vi "Tosca-Analog Input Thread.vi"() -> ()   [LabVIEW 2020]
uses:
  Typedefs/Tosca-AI Live Controls.ctl
  Typedefs/Tosca-AI Stream Controls.ctl
  Typedefs/Tosca-AI UI State.ctl
  Typedefs/Tosca-AI Plot Properties.ctl
  Typedefs/Tosca-AI Control Queue Data.ctl
  Typedefs/Tosca-AI.ctl
  epl-vi-lib/TCP VIs/TCP Params.ctl
  epl-vi-lib/PXI DAQ VIs/AIDI/Typedefs/AIDI-Action.ctl
  62174e53-180b-4f65-acbd-20ff4249b710.vi
  epl-vi-lib/Utility VIs/Comparison VIs/Arrays Equal (STR).vi
  Sub VIs/Tosca-Globals.vi
panel:
  out "Digital":dbl[][](graph)
  in  "More":bool=TRUE
  out "Analog":dbl[][](graph)
  in  "Trace":bool=TRUE caption="All"
  in  "Vscale":dbl=1e-09 min=1e-09 max=10.0 format="%.0pV"
  in  "Stack":bool
  in  "Vscale":bool
  out "Load":dbl(slide) caption="5 ms" scale=0.0..1.0
  in  "Status":string
  out "scale":dbl format="1div = %.0ps"
  out "recording":bool
  in  "stream":T1
  in  "Record":bool
  in  "live":T2
  in  "finished":errorcluster
  in  "History (s)":dbl=5.0
  in  "T (ms)":dbl=500.0 caption="Frame size (ms)"
  in  "Legend":i32(listbox)
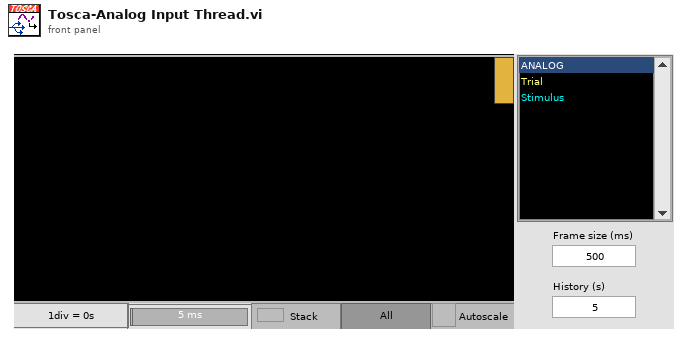
[diagram p1: front panel]
types:
  T1 = typedef "Tosca-AI Stream Controls.ctl" = cluster{"record":bool, "stem":string}
  T2 = typedef "Tosca-AI Live Controls.ctl" = cluster{"Global":cluster{"stack":bool, "auto":bool, "max":dbl}, "DI":bool[], "AI":cluster{"visible":bool, "auto":bool, "max":dbl}[], "plot AI":bool, "plot DI":bool}
  T3 = typedef "TCP Params.ctl" = cluster{"IP Address":string, "Port":i32}
  T4 = typedef "Tosca-AI.ctl" = cluster{"active":bool, "Fs":dbl, "AI":string[], "DI":string[]}
  T5 = typedef "Tosca-AI Control Queue Data.ctl" = cluster{"AI":T4, "History (s)":dbl, "T (ms)":dbl}
  T6 = typedef "Tosca-AI UI State.ctl" = cluster{"map":T7[], "running":bool, "locked":bool, "Global":cluster{"stack":bool, "auto":bool, "max":dbl}, "SelAI":i32, "first AI":i32, "plot AI":bool, "plot DI":bool, "next":string}
  T7 = typedef "Tosca-AI Plot Properties.ctl" = cluster{"graph":refnum<vi>, "plot":i32, "color":u32, "auto":bool, "visible":bool, "name":string, "digital?":bool, "max":dbl}
  T8 = cluster{"Run":refnum<user-event>, "Record":refnum<user-event>, "Stop":refnum<user-event>}
  T9 = enum8{"Enabled", "Disabled", "Disabled and Grayed Out"}
  T10 = enum16{"Sticks Top/Left", "Sticks Bottom/Right", "Proportional"}
  T11 = typedef "LVPoint32TypeDef.ctl" = cluster{"Horizontal":i32, "Vertical":i32}
  T12 = cluster{"AI":T4, "History (s)":dbl, "T (ms)":dbl}
  T13 = typedef "AIDI-Action.ctl" = enum16{"Configure", "Initialize", "Start", "Read", "Clean up", "Init & Start", "Config & Test", "Position", "Skip"}
  T14 = typedef "Tosca-AI Plot State.ctl" = cluster{"offset":i32, "nseg":i32, "nblank":i32, "npts":i32, "AI max":dbl[][], "stream":bool, "filename":string, "filenum":i32, "indicator":i32, "last ind":bool, "dig ind":bool, "nstream":i32, "istream":i32, "file":refnum<file>, "AI order":i32[], "DI order":i32[]}
  T15 = cluster{"Elapsed time (ms)":dbl, "filename":string}
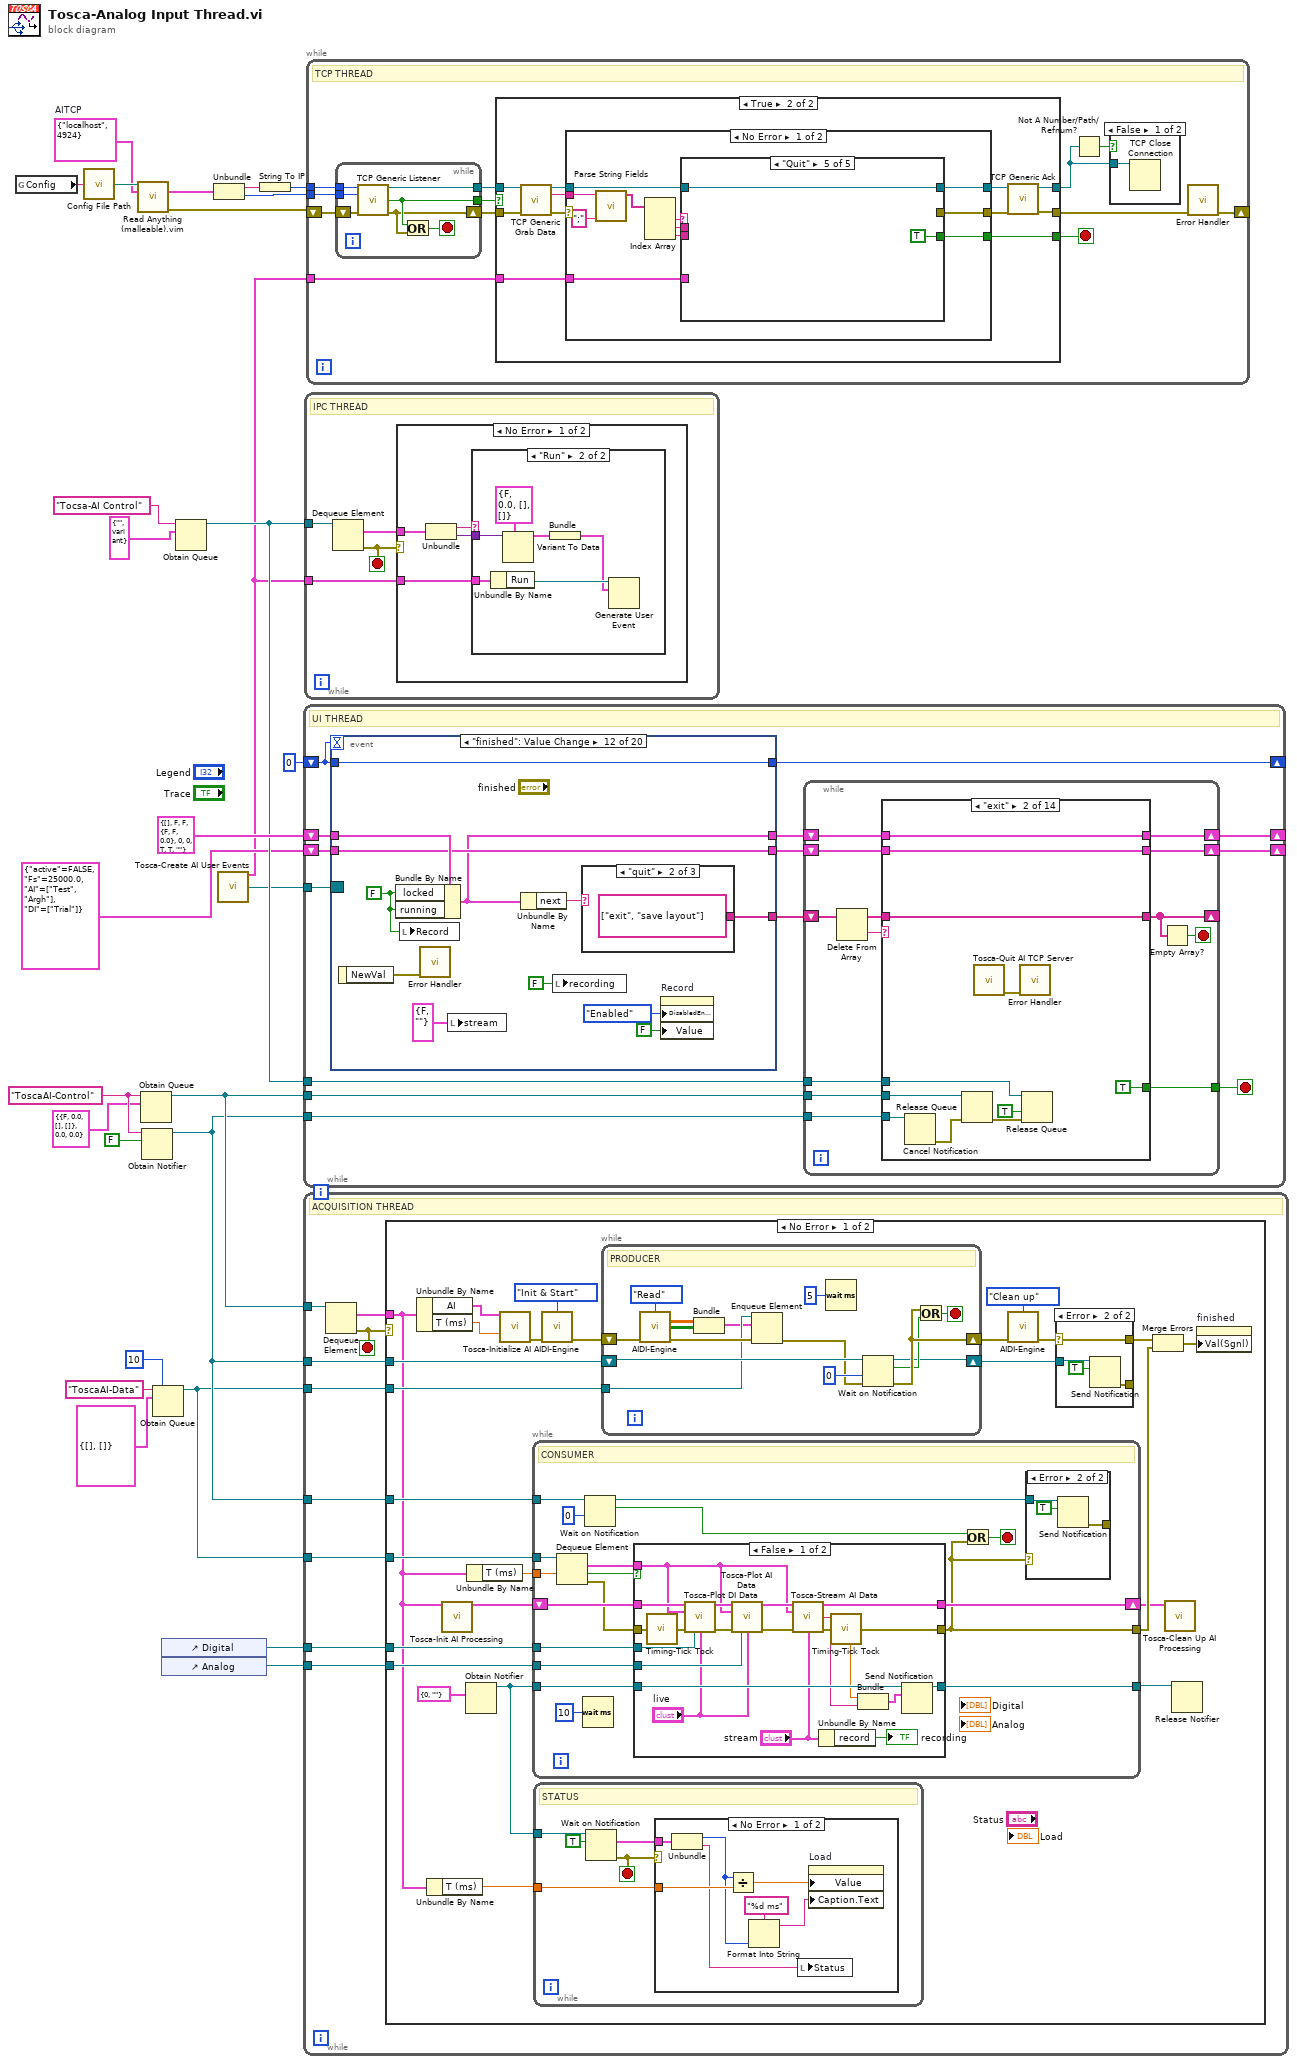
[diagram p0: block diagram]
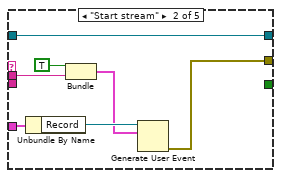
[diagram p5: hidden frame]
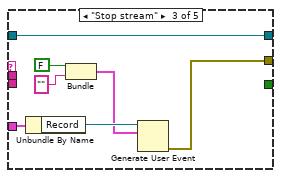
[diagram p6: hidden frame]
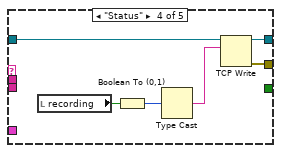
[diagram p7: hidden frame]
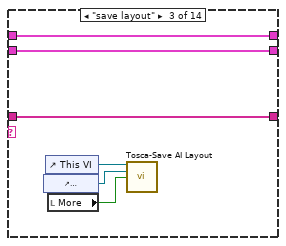
[diagram p12: hidden frame]
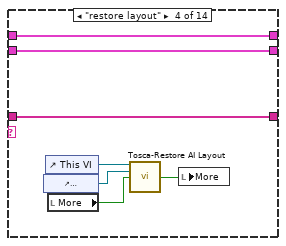
[diagram p13: hidden frame]
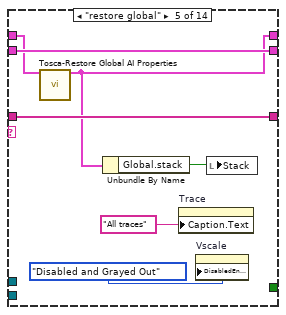
[diagram p14: hidden frame]
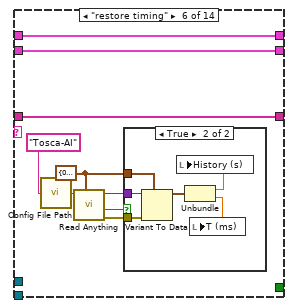
[diagram p15: hidden frame]
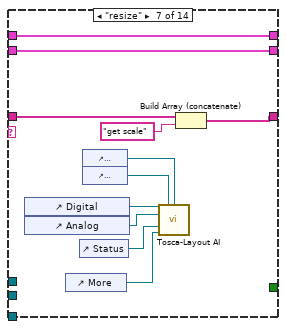
[diagram p17: hidden frame]
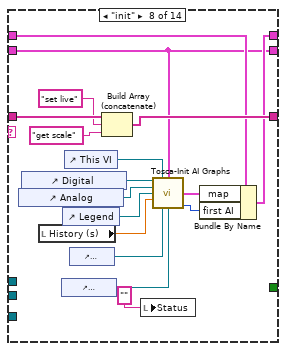
[diagram p18: hidden frame]
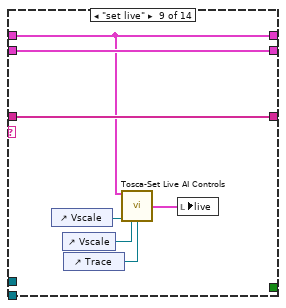
[diagram p19: hidden frame]
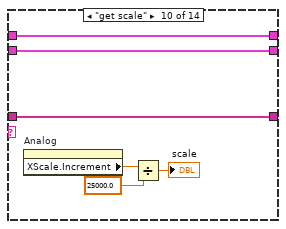
[diagram p20: hidden frame]
diagram:
  w3 = T3 {"IP Address"="localhost", "Port"=4924}  # AITCP
  w24 = "ToscaAI-Control" ("name (unnamed)")
  n1 = global read "Tosca-Globals.vi" "Config"() -> (w5:string)
  n2 = call "Config File Path.vi"("AppName"=w5) -> ("Default config file name"=w4:path)
  n3 = call "Read Anything (malleable).vim"("Config file path"=w4, "Options in"=w3) -> ("Options out"=w2:T3, "error out"=w1:errorcluster)  [unwired: 10 in, 2 out]
  n4 = Obtain Queue(name (unnamed)=w24, element data type=T5 {"AI"={"active"=FALSE, "Fs"=0.0, "AI"=[], "DI"=[]}, "History (s)"=0.0, "T (ms)"=0.0} ("output cluster")) -> (queue out=w25:refnum<queue>)  [unwired: 3 in, 2 out]
  n5 = Obtain Notifier(name (unnamed)=w24, notification data type=FALSE) -> (notifier out=w18:refnum<notifier>)  [unwired: 2 in, 2 out]
  n6 = Obtain Queue(max queue size (-1, unlimited)=10, name (unnamed)="ToscaAI-Data", element data type=cluster{dbl[][], bool[][]} {[], []}) -> (queue out=w17:refnum<queue>)  [unwired: 2 in, 2 out]
  n7 = control-ref of="Digital"() -> (w15:refnum<vi>)
  n8 = control-ref of="Analog"() -> (w20:refnum<vi>)
  n9 = Obtain Queue(name (unnamed)="Tocsa-AI Control", element data type=cluster{"Action":string, "Data":variant} {"Action"="", "Data"=variant} ("Data")) -> (queue out=w12:refnum<queue>)  [unwired: 3 in, 2 out]
  n10 = Unbundle(w2) -> ("IP Address"=w8:string, "Port"=w6:i32)
  n11 = call "Tosca-Create AI User Events.vi"() -> ("events"=w9:T8, "Event Registration Refnum"=w10:refnum<event-registration>)  [unwired: 14 in]
  n12 = String To IP(1:w8) -> (0:w7:u32)
  n13 = while {
    shift-right: [w40] -> _
    shift-left: 0 -> [w41]
    shift-right: [w35] -> _
    shift-left: T6 {"map"=[], "running"=FALSE, "locked"=FALSE, "Global"={"stack"=FALSE, "auto"=FALSE, "max"=0.0}, "SelAI"=0, "first AI"=0, "plot AI"=TRUE, "plot DI"=TRUE, "next"=""} ("state") -> [w37]
    tunnel: w25 -> [w31]
    shift-right: [w32] -> _
    shift-left: T4 {"active"=FALSE, "Fs"=25000.0, "AI"=["Test", "Argh"], "DI"=["Trial"]} ("AI") -> [w34]
    tunnel: w18 -> [w30]
    tunnel: w12 -> [w29]
    tunnel: w10 -> [w28]
    stop <- w38 stop-if-true
    # "UI THREAD"
    n14 = event shown="[11] \"finished\": Value Change" {
      selector: w28 -> [_ _ _ _ _ _ _ _ _ _ _ _ _ _ _ _ _ _ _ _]
      dyn-events: _ -> [_ _ _ _ _ _ _ _ _ _ _ _ _ _ _ _ _ _ _ _]
      timeout: w41 -> [_ _ _ _ _ _ _ _ _ _ _ _ _ _ _ _ _ _ _ _]
      tunnel: w41 -> [_ w187 w193 w197 w214 w221 w228 w236 w251 w279 w285 w310 w321 w327 w333 w342 w354 w371 w386 w393]
      tunnel: [-1 w187 w193 w197 w214 w221 w228 w236 w251 w279 w285 w310 w321 w327 w333 w342 w354 w371 w386 w393] -> w40
      tunnel: [string[] ["init", "restore global", "restore timing", "resize", "restore layout"] w186 string[] ["save layout", "resize"] string[] ["save layout", "resize"] string[] ["save layout"] string[] ["set live"] _ _ w244 _ w283 w303 string[] ["set live"] string[] ["set live"] string[] ["set live"] _ _ w370 _ w388] -> w39
      tunnel: w37 -> [w179 w183 w191 w195 w200 w219 w223 w231 w246 w265 w281 w309 w320 w324 w330 w341 w353 w362 w385 w390]
      tunnel: [w179 w183 w191 w195 w200 w218 w223 w230 w245 w265 w280 w305 w314 w322 w329 w341 w353 w362 w383 w390] -> w36
      tunnel: w34 -> [w178 w184 w190 w194 w198 w220 w222 w229 w250 w266 w282 w308 w319 w326 w332 w340 w352 w365 w384 w392]
      tunnel: [w178 w184 w190 w194 w198 w220 w222 w229 w250 w266 w282 w308 w319 w326 w332 w340 w352 w364 w384 w392] -> w33
      event Timeout {
        n15 = event-data() -> ()  [unwired: 1 in, 1 out]
        n16 = property on="Record" class="Bool (strict)"("DisabledEnum"=T9."Enabled" ("Disabled"), "Value"=FALSE ("Record")) -> ()  [unwired: 2 in, 2 out]
        n17 = local write "recording"(FALSE ("recording")) -> ()
      }
      event Panel Close? {
        n18 = event-data() -> ()  [unwired: 1 in, 1 out]
        n19 = Unbundle By Name(w183) -> ("running"=w182:bool)
        n20 = case shown="True" w182 {
          tunnel: [string[] ["exit", "save layout"] string[] ["stop&quit"]] -> w186
          frame False {
          }
          frame True {
          }
        }
        n21 = event-data("Discard?"=TRUE) -> ()  [unwired: 1 in, 1 out]
      }
      event Panel Resize {
        n22 = event-data() -> ()  [unwired: 1 in, 1 out]
      }
      event Pane Size {
        n23 = event-data() -> ()  [unwired: 1 in, 1 out]
      }
      event "More": Value Change {
        n24 = event-data() -> ()  [unwired: 1 in, 1 out]
        n25 = control-ref of="This VI"() -> (w208:refnum<vi>)
        n26 = property on="Splitter" class="Splitter"("Sizing"=T10."Sticks Top/Left") -> (error out=w205:errorcluster)  [unwired: 2 in, 1 out]
        n27 = Select(t=157, s="More", f=-157) -> (s? t:f=w212:i32)
        n28 = call "Get Window Width.vi"("VI in"=w208, "error in (no error)"=w205) -> ("VI out"=w209:refnum<vi>, "Width"=w207:i16, "error out"=w201:errorcluster)  [unwired: 11 in]
        n29 = Add(x=w207, y=w212) -> (x+y=w206:i32)
        n30 = call "Set Window Width.vi"("VI in"=w209, "Width"=w206, "error in (no error)"=w201) -> ("error out"=w203:errorcluster)  [unwired: 11 in, 1 out]
        n31 = property on="Splitter" class="Splitter"(error in=w203, "Sizing"=T10."Sticks Bottom/Right") -> ()  [unwired: 1 in, 2 out]
      }
      event "Legend": Double Click {
        n32 = event-data() -> ("Row"=w217:i32)  [unwired: 1 in]
        n33 = control-ref of="Legend"() -> (w216:refnum<vi>)
        n34 = call "Tosca-Process AI Double Click.vi"("state in"=w219, "Legend"=w216, "Row"=w217) -> ("state out"=w218:T6)  [unwired: 12 in]
      }
      event "Legend": Shortcut Menu Activation? {
        n35 = event-data() -> ("CtlRef"=w225:refnum<vi>, "MenuRef"=w226:refnum<k9>, "Coords"=w227:T11)  [unwired: 1 in]
        n36 = call "Tosca-Create AI Legend Context Menu.vi"("ListBox in"=w225, "MenuRef"=w226, "Coords"=w227) -> ("discard"=w224:bool)  [unwired: 12 in]
        n37 = event-data("Discard?"=w224) -> ()  [unwired: 1 in, 1 out]
      }
      event "Legend": Shortcut Menu Selection (User) {
        n38 = event-data() -> ("ItemTag"=w235:string)  [unwired: 1 in]
        n39 = Match Pattern(string=w235, regular expression="cmColor_") -> (match substring=w233:string, after substring=w232:string)  [unwired: 1 in, 2 out]
        n40 = case shown="\"cmColor_\"" w233 {
          tunnel: w232 -> [_ w243]
          tunnel: w231 -> [w237 w241]
          tunnel: [w237 w240] -> w230
          frame "", Default {
          }
          frame "cmColor_" {
            n41 = control-ref of="Legend"() -> (w238:refnum<vi>)
            n42 = Decimal String To Number(string=w243) -> (number=w242:i32)  [unwired: 2 in, 1 out]
            n43 = control-ref of="This VI"() -> (w239:refnum<vi>)
            n44 = call "Tosca-Process AI Color Change.vi"("state in"=w241, "Legend"=w238, "VI in"=w239, "Row"=w242) -> ("state out"=w240:T6)  [unwired: 11 in]
          }
        }
      }
      event "Legend": Value Change {
        n45 = event-data() -> ("NewVal"=w247:i32)  [unwired: 1 in]
        n46 = Unbundle By Name(w246) -> ("first AI"=w249:i32)
        n47 = Greater Or Equal?(x=w247, y=w249) -> (x >= y?=w248:bool)
        n48 = case shown="True" w248 {
          tunnel: w246 -> [w252 w256]
          tunnel: w247 -> [_ w255]
          tunnel: [w252 w254] -> w245
          tunnel: [_ string[] ["set live"]] -> w244
          frame False {
          }
          frame True {
            n49 = Bundle By Name(cluster=w256, "SelAI"=w255) -> (w254:T6)
          }
        }
      }
      event Shortcut Menu Activation? {
        n50 = event-data() -> ("MenuRef"=w278:refnum<k9>)  [unwired: 1 in]
        n51 = Unbundle By Name(w265) -> ("running"=w268:bool, "plot AI"=w261:bool)
        n52 = Delete Menu Items(9:w278) -> (3:w275:refnum<k9>)  [unwired: 3 in, 1 out]
        n53 = Unbundle By Name(w265) -> ("locked"=w272:bool)
        n54 = Not(x=w272) -> (.not. x?=w271:bool)
        n55 = Select(t="cmStop", s=w268, f="cmRun") -> (s? t:f=w264:string)
        n56 = Select(t="cmPause", s=w261, f="cmPlot") -> (s? t:f=w259:string)
        n57 = Build Array(w264, "APP_SEPARATOR" ("element"), w259) -> (w267:string[])
        n58 = Insert Menu Items(7:w267, 8:string[] ["Run", "-", "Plot"] ("item names"), 9:w275) -> (0:w274:errorcluster, 3:w273:refnum<k9>)  [unwired: 3 in, 1 out]
        n59 = Set Menu Item Info(6:w268, 7:w264, 8:w274, 9:w271, 11:w273) -> (0:w262:errorcluster, 3:w263:refnum<k9>)  [unwired: 2 in]
        n60 = event-data("Discard?"=FALSE) -> ()  [unwired: 1 in, 1 out]
        n61 = Set Menu Item Info(6:w261, 7:w259, 8:w262, 11:w263) -> ()  [unwired: 3 in, 2 out]
      }
      event Shortcut Menu Selection (User) {
        n62 = event-data() -> ("ItemTag"=w284:string)  [unwired: 1 in]
        n63 = case shown="\"cmRun\"" w284 {
          tunnel: [_ string[] ["run", "init"] string[] ["stop"] string[] ["set live"] string[] ["set live"]] -> w283
          tunnel: w281 -> [w286 w287 w289 w293 w297]
          tunnel: [w286 w287 w289 w292 w296] -> w280
          frame "", Default {
          }
          frame "cmRun" {
          }
          frame "cmStop" {
          }
          frame "cmPlot" {
            w291 = TRUE ("plot AI")
            n64 = Bundle By Name(cluster=w293, "plot AI"=w291, "plot DI"=w291) -> (w292:T6)
          }
          frame "cmPause" {
            w295 = FALSE ("plot AI")
            n65 = Bundle By Name(cluster=w297, "plot AI"=w295, "plot DI"=w295) -> (w296:T6)
          }
        }
      }
      event "finished": Value Change {
        w302 = FALSE ("running")
        n66 = event-data() -> ("NewVal"=w307:errorcluster)  [unwired: 1 in]
        n67 = Bundle By Name(cluster=w309, "locked"=w302, "running"=w302) -> (w305:T6)
        n68 = local write "Record"(w302) -> ()
        n69 = call "Error Handler.vi"("error in (no error)"=w307) -> ()  [unwired: 12 in, 3 out]
        n70 = local write "stream"(T1 {"record"=FALSE, "stem"=""} ("stream")) -> ()
        n71 = Unbundle By Name(w305) -> ("next"=w304:string)
        n72 = local write "recording"(FALSE ("recording")) -> ()
        n73 = case shown="\"quit\"" w304 {
          tunnel: [_ string[] ["exit", "save layout"] string[] ["run", "init"]] -> w303
          frame "", Default {
          }
          frame "quit" {
          }
          frame "restart" {
          }
        }
        n74 = property on="Record" class="Bool (strict)"("DisabledEnum"=T9."Enabled" ("Disabled"), "Value"=FALSE ("Record")) -> ()  [unwired: 2 in, 2 out]
      }
      event "Stack": Value Change {
        n75 = event-data() -> ()  [unwired: 1 in, 1 out]
        n76 = Bundle By Name(cluster=w320, "Global.stack"="Stack") -> (w314:T6)
        n77 = Unbundle By Name(w314) -> ("Global"=w313:cluster{"stack":bool, "auto":bool, "max":dbl})
        n78 = call "Config File Path.vi"("AppName"="Tosca-AI") -> ("Default config file name"=w316:path)
        n79 = call "Write Anything.vi"("Anything"=w313, "Path (dialog)"=w316) -> ()  [unwired: 8 in, 2 out]
      }
      event "Vscale": Value Change {
        n80 = event-data() -> ()  [unwired: 1 in, 1 out]
        n81 = call "Tosca-Process Autoscale Change.vi"("state in"=w324, "autoscale"="Vscale") -> ("state out"=w322:T6)  [unwired: 13 in]
      }
      event "Vscale": Value Change {
        n82 = event-data() -> ()  [unwired: 1 in, 1 out]
        n83 = call "Tosca-Process Max Change.vi"("state in"=w330, "max"="Vscale") -> ("state out"=w329:T6)  [unwired: 13 in]
      }
      event "T (ms)", "History (s)": Value Change {
        n84 = event-data() -> ()  [unwired: 1 in, 1 out]
        n85 = Bundle("History (s)"="History (s)", "T (ms)"="T (ms)") -> (w335:cluster{"History (s)":dbl, "T (ms)":dbl})  [unwired: 1 in]
        n86 = call "Config File Path.vi"("AppName"="Tosca-AI") -> ("Default config file name"=w336:path)
        n87 = call "Write Anything.vi"("Section Name (Name of \"Anything\")"="Timing" ("Section Name (Name of \"Anything\")"), "Anything"=w335, "Path (dialog)"=w336) -> ()  [unwired: 7 in, 2 out]
      }
      event "Record": Value Change {
        n88 = event-data() -> ()  [unwired: 1 in, 1 out]
        n89 = Format Date/Time String(time format string (%c)="_%y%b%d_%H%M%S") -> (date/time string=w351:string)  [unwired: 2 in]
        n90 = Concatenate Strings("ToscaAI" ("string"), w351) -> (w348:string)
        n91 = Build Path(base path=path "C:/Data/Tosca/Data/AI", name or relative path=w348) -> (appended path=w346:path)
        n92 = Path To String(path=w346) -> (string=w344:string)
        n93 = Bundle("Record"="Record", w344) -> (w343:cluster{"Record":bool, string})  [unwired: 1 in]
        n94 = local write "stream"(w343) -> ()
      }
      event User Event {
        n95 = event-data() -> ("AI.Fs"=w368:dbl, "AI.AI"=w359:string[], "AI.DI"=w357:string[], "AI"=w363:T4)  [unwired: 1 in]
        n96 = Unbundle By Name(w365) -> ("Fs"=w369:dbl, "AI"=w360:string[], "DI"=w358:string[])
        n97 = Not Equal?(x=w369, y=w368) -> (x != y?=w367:bool)
        n98 = call-poly "Arrays Equal.vi"("Array 2"=w359, "Array 1"=w360) -> ("arrays equal?"=w356:bool)
        n99 = call-poly "Arrays Equal.vi"("Array 2"=w357, "Array 1"=w358) -> ("arrays equal?"=w355:bool)
        n100 = Unbundle By Name(w362) -> ("running"=w361:bool)
        n101 = Compound Arithmetic op=OR(w367, invert w356, invert w355) -> (w366:bool)
        n102 = case shown="True" w366 {
          tunnel: [_ w374] -> w370
          tunnel: w365 -> [w372 _]
          tunnel: [w372 w375] -> w364
          tunnel: w363 -> [_ w375]
          tunnel: w361 -> [_ w373]
          frame False {
          }
          frame True {
            n103 = case shown="False" w373 {
              tunnel: [string[] ["run", "init"] string[] ["stop&resart"]] -> w374
              frame False {
              }
              frame True {
              }
            }
          }
        }
      }
      event User Event {
        n104 = event-data() -> ("record"=w378:bool, "stem"=w379:string)  [unwired: 1 in]
        n105 = Bundle("record"=w378, "stem"=w379) -> (w382:cluster{"record":bool, "stem":string})  [unwired: 1 in]
        n106 = local write "stream"(w382) -> ()
        n107 = property on="Record" class="Bool (strict)"("Value"=TRUE ("Record"), "DisabledEnum"=T9."Disabled and Grayed Out" ("Disabled")) -> ()  [unwired: 2 in, 2 out]
        n108 = Bundle By Name(cluster=w385, "locked"=w378) -> (w383:T6)
      }
      event User Event {
        n109 = event-data() -> ("exit"=w387:bool)  [unwired: 1 in]
        n110 = local write "stream"(T1 {"record"=FALSE, "stem"=""} ("stream")) -> ()
        n111 = Unbundle By Name(w390) -> ("running"=w389:bool)
        n112 = case shown="True" w387 {
          tunnel: w389 -> [_ w395]
          tunnel: [_ w394] -> w388
          frame False {
          }
          frame True {
            n113 = case shown="False" w395 {
              tunnel: [string[] ["exit", "save layout"] string[] ["stop&quit"]] -> w394
              frame False {
              }
              frame True {
              }
            }
          }
        }
      }
    }
    n114 = while {
      shift-right: [w51] -> _
      shift-left: w39 -> [w54]
      tunnel: [w49] -> w38
      shift-right: [w47] -> w35
      shift-left: w36 -> [w48]
      shift-right: [w45] -> w32
      shift-left: w33 -> [w46]
      tunnel: w31 -> [w44]
      tunnel: w30 -> [w43]
      tunnel: w29 -> [w42]
      stop <- w50 stop-if-true
      n115 = Delete From Array(array=w54) -> (deleted portion=w53:string, array with subset deleted=w52:string[])  [unwired: 2 in]
      n116 = case shown="\"exit\"" w53 {
        tunnel: w52 -> [w57 w68 w74 w81 w88 w97 w114 w131 w138 w144 w155 w160 w167 w174]
        tunnel: [w57 w68 w74 w81 w88 w97 w108 w126 w138 w144 w155 w160 w167 w174] -> w51
        tunnel: [_ TRUE _ _ _ _ _ _ _ _ _ _ _ _] -> w49
        tunnel: [w56 w66 w73 w80 w85 w96 w105 w122 w136 w140 w152 w159 w162 w169] -> w47
        tunnel: w48 -> [w56 w66 w73 w80 w86 w96 w105 w123 w136 w140 w154 w159 w166 w173]
        tunnel: w46 -> [w55 w65 w69 w75 w87 w95 w104 w118 w137 w139 w148 w158 w165 w172]
        tunnel: [w55 w65 w69 w75 w87 w95 w104 w118 w137 w139 w148 w158 w165 w172] -> w45
        tunnel: w44 -> [_ w64 _ _ _ _ _ _ _ _ w153 _ _ _]
        tunnel: w43 -> [_ w63 _ _ _ _ _ _ _ _ w150 w157 w164 w171]
        tunnel: w42 -> [_ w60 _ _ _ _ _ _ _ _ _ _ _ _]
        frame "", Default {
        }
        frame "exit" {
          n117 = Cancel Notification(0:w63) -> (11:w62:errorcluster)  [unwired: 1 in, 2 out]
          n118 = Release Queue(queue=w64, error in (no error)=w62) -> (error out=w61:errorcluster)  [unwired: 1 in, 2 out]
          n119 = call "Tosca-Quit AI TCP Server.vi"() -> ("error out"=w58:errorcluster)  [unwired: 15 in]
          n120 = call "Error Handler.vi"("error in (no error)"=w58) -> ()  [unwired: 12 in, 3 out]
          n121 = Release Queue(queue=w60, force destroy? (F)=TRUE, error in (no error)=w61) -> ()  [unwired: 3 out]
        }
        frame "save layout" {
          n122 = control-ref of="GraphSplitter"() -> (w71:refnum<vi>)
          n123 = control-ref of="This VI"() -> (w72:refnum<vi>)
          n124 = local read "More"() -> (w70:bool)
          n125 = call "Tosca-Save AI Layout.vi"("VI in"=w72, "GraphSplitter"=w71, "More"=w70) -> ()  [unwired: 12 in, 1 out]
        }
        frame "restore layout" {
          n126 = control-ref of="GraphSplitter"() -> (w78:refnum<vi>)
          n127 = control-ref of="This VI"() -> (w79:refnum<vi>)
          n128 = local read "More"() -> (w77:bool)
          n129 = call "Tosca-Restore AI Layout.vi"("VI in"=w79, "GraphSplitter"=w78, "more in"=w77) -> ("more out"=w76:bool)  [unwired: 11 in, 1 out]
          n130 = local write "More"(w76) -> ()
        }
        frame "restore global" {
          n131 = call "Tosca-Restore Global AI Properties.vi"("state in"=w86) -> ("state out"=w85:T6)  [unwired: 14 in]
          n132 = Unbundle By Name(w85) -> ("Global.stack"=w84:bool)
          n133 = property on="Trace" class="Bool"("Caption.Text"="All traces") -> ()  [unwired: 2 in, 2 out]
          n134 = property on="Vscale" class="DigNum (strict)"("DisabledEnum"=T9."Disabled and Grayed Out" ("Disabled")) -> ()  [unwired: 2 in, 2 out]
          n135 = local write "Stack"(w84) -> ()
        }
        frame "restore timing" {
          w89 = cluster{dbl, dbl} {0.0, 0.0}
          n136 = call "Config File Path.vi"("AppName"="Tosca-AI") -> ("Default config file name"=w93:path)
          n137 = call "Read Anything.vi"("Type of Anything"=w89, "Path (dialog)"=w93) -> ("Error Out"=w90:errorcluster, "Found?"=w91:bool, "Anything"=w92:variant)  [unwired: 7 in]
          n138 = case shown="True" w91 {
            tunnel: w92 -> [_ w102]
            tunnel: w90 -> [_ w103]
            tunnel: w89 -> [_ w101]
            frame False {
            }
            frame True {
              n139 = Variant To Data(error in=w103, type=w101, Variant=w102) -> (data=w100:cluster{dbl, dbl})  [unwired: 1 out]
              n140 = Unbundle(w100) -> (w99:dbl, w98:dbl)
              n141 = local write "History (s)"(w99) -> ()
              n142 = local write "T (ms)"(w98) -> ()
            }
          }
        }
        frame "resize" {
          n143 = control-ref of="Digital"() -> (w106:refnum<vi>)
          n144 = control-ref of="Analog"() -> (w113:refnum<vi>)
          n145 = control-ref of="More"() -> (w109:refnum<vi>)
          n146 = control-ref of="Status"() -> (w110:refnum<vi>)
          n147 = control-ref of="AnalogPane"() -> (w112:refnum<vi>)
          n148 = control-ref of="DigitalPane"() -> (w111:refnum<vi>)
          n149 = call "Tosca-Layout AI.vi"("Digital"=w106, "DigitalPane"=w111, "AnalogPane"=w112, "Analog"=w113, "Status"=w110, "More"=w109) -> ()  [unwired: 10 in]
          n150 = Build Array (concatenate)(w114, "get scale") -> (w108:string[])
        }
        frame "init" {
          n151 = control-ref of="Analog"() -> (w129:refnum<vi>)
          n152 = control-ref of="Digital"() -> (w124:refnum<vi>)
          n153 = local read "History (s)"() -> (w127:dbl)
          n154 = control-ref of="GraphSplitter"() -> (w119:refnum<vi>)
          n155 = control-ref of="Legend"() -> (w128:refnum<vi>)
          n156 = control-ref of="This VI"() -> (w115:refnum<vi>)
          n157 = control-ref of="DigitalPane"() -> (w120:refnum<vi>)
          n158 = Build Array (concatenate)(w131, "set live" ("element"), "get scale") -> (w126:string[])
          n159 = local write "Status"("" ("Status")) -> ()
          n160 = call "Tosca-Init AI Graphs.vi"("Digital"=w124, "VI in"=w115, "AI"=w118, "Analog"=w129, "Legend"=w128, "History (s)"=w127, "Pane in"=w120, "Splitter"=w119) -> ("plot map"=w121:T7[], "first AI"=w116:i32)  [unwired: 6 in]
          n161 = Bundle By Name(cluster=w123, "map"=w121, "first AI"=w116) -> (w122:T6)
        }
        frame "set live" {
          n162 = control-ref of="Vscale"() -> (w134:refnum<vi>)
          n163 = control-ref of="Vscale"() -> (w133:refnum<vi>)
          n164 = control-ref of="Trace"() -> (w132:refnum<vi>)
          n165 = call "Tosca-Set Live AI Controls.vi"("state"=w136, "Auto"=w134, "Vscale"=w133, "Trace"=w132) -> ("Controls"=w135:T2)  [unwired: 11 in]
          n166 = local write "live"(w135) -> ()
        }
        frame "get scale" {
          n167 = property on="Analog" class="WFGraph (strict)"() -> ("XScale.Increment"=w143:dbl)  [unwired: 2 in, 2 out]
          n168 = Divide(x=w143, y=25000.0) -> (x/y=→"scale":dbl)
        }
        frame "run" {
          n169 = Cancel Notification(0:w150) -> (11:w149:errorcluster)  [unwired: 1 in, 2 out]
          n170 = local read "History (s)"() -> (w146:dbl)
          n171 = local read "T (ms)"() -> (w145:dbl)
          n172 = Bundle("AI"=w148, "History (s)"=w146, "T (ms)"=w145) -> (w147:T12)  [unwired: 1 in]
          n173 = Bundle By Name(cluster=w154, "running"=TRUE) -> (w152:T6)
          n174 = Enqueue Element(queue=w153, element=w147, error in (no error)=w149) -> ()  [unwired: 1 in, 3 out]
        }
        frame "stop" {
          n175 = Send Notification(notification=TRUE, notifier=w157) -> ()  [unwired: 1 in, 2 out]
        }
        frame "stop&quit" {
          n176 = Send Notification(notification=TRUE, notifier=w164) -> ()  [unwired: 1 in, 2 out]
          n177 = Bundle By Name(cluster=w166, "next"="quit") -> (w162:T6)
        }
        frame "stop&restart" {
          n178 = Send Notification(notification=TRUE, notifier=w171) -> ()  [unwired: 1 in, 2 out]
          n179 = Bundle By Name(cluster=w173, "next"="restart") -> (w169:T6)
        }
      }
      n180 = Empty Array?(array=w51) -> (empty?=w50:bool)
    }
  }
  n181 = while {
    tunnel: w25 -> [w406]
    tunnel: w18 -> [w403]
    tunnel: w17 -> [w402]
    tunnel: w20 -> [w401]
    tunnel: w18 -> [w400]
    tunnel: w17 -> [w399]
    tunnel: w15 -> [w398]
    stop <- w405 stop-if-true
    # "ACQUISITION THREAD"
    n182 = Dequeue Element(queue=w406) -> (element=w404:T5, error out=w405:errorcluster)  [unwired: 2 in, 2 out]
    n183 = case shown="No Error" w405 {
      tunnel: w404 -> [w407 _]
      tunnel: w403 -> [w432 _]
      tunnel: w402 -> [w411 w510]
      tunnel: w401 -> [w430 _]
      tunnel: w400 -> [w429 _]
      tunnel: w399 -> [w428 _]
      tunnel: w398 -> [w423 _]
      frame No Error {
        n184 = Unbundle By Name(w407) -> ("AI"=w413:T4, "T (ms)"=w412:dbl)
        n185 = Unbundle By Name(w407) -> ("T (ms)"=w425:dbl)
        n186 = call "Tosca-Init AI Processing.vi"("Queue data"=w407) -> ("state"=w431:T14)  [unwired: 14 in]
        n187 = Obtain Notifier(notification data type=cluster{"elapsed":u32, "name":string} {"elapsed"=0, "name"=""}) -> (notifier out=w427:refnum<notifier>)  [unwired: 3 in, 2 out]
        n188 = Unbundle By Name(w407) -> ("T (ms)"=w424:dbl)
        n189 = call "Tosca-Initialize AI.vi"("AI"=w413, "T (ms)"=w412) -> ("error out"=w416:errorcluster)  [unwired: 13 in]
        n190 = while {
          shift-right: [w454] -> w419
          shift-left: w431 -> [w469]
          tunnel: w430 -> [w466]
          tunnel: w429 -> [w465]
          tunnel: w428 -> [w464]
          tunnel: w424 -> [w459]
          tunnel: w427 -> [w458]
          tunnel: [w457] -> w426
          tunnel: w423 -> [w456]
          tunnel: [w453] -> w420
          stop <- w470 stop-if-true
          # "CONSUMER"
          n191 = Dequeue Element(queue=w464, timeout in ms (-1)=w459) -> (element=w462:cluster{dbl[][], bool[][]}, timed out?=w461:bool, error out=w460:errorcluster)  [unwired: 1 in, 1 out]
          n192 = Wait (ms)(milliseconds to wait=u32 10) -> ()  [unwired: 1 out]
          n193 = Wait on Notification(notifier=w465, timeout in ms (-1)=0) -> (notifier out=w455:refnum<notifier>, notification=w468:bool)  [unwired: 2 in, 2 out]
          n194 = case shown="False" w461 {
            tunnel: w469 -> [w483 w497]
            tunnel: [w480 w497] -> w454
            tunnel: w462 -> [w477 _]
            tunnel: [w490 w496] -> w453
            tunnel: w460 -> [w494 w496]
            tunnel: w466 -> [w493 _]
            tunnel: w458 -> [w492 w495]
            tunnel: [w491 w495] -> w457
            tunnel: w456 -> [w482 _]
            frame False {
              n195 = call "Timing-Tick Tock.vi"("error in (no error)"=w494) -> ("error out"=w487:errorcluster)  [unwired: 5 in, 1 out]
              n196 = call "Tosca-Plot DI Data.vi"("state in"=w483, "Data"=w477, "error in (no error)"=w487, "Digital"=w482, "Controls"="live") -> ("state out"=w484:T14, "error out"=w486:errorcluster)  [unwired: 9 in]
              n197 = call "Tosca-Plot AI Data.vi"("state in"=w484, "Data"=w477, "error in (no error)"=w486, "Analog"=w493, "Controls"="live") -> ("state out"=w478:T14, "error out"=w481:errorcluster)  [unwired: 9 in]
              n198 = call "Tosca-Stream AI Data.vi"("state in"=w478, "Data"=w477, "error in (no error)"=w481, "stream"="stream") -> ("state out"=w480:T14, "filename"=w476:string, "error out"=w479:errorcluster)  [unwired: 9 in]
              n199 = Unbundle By Name("stream") -> ("record"=→"recording":bool)
              n200 = call "Timing-Tick Tock.vi"("error in (no error)"=w479) -> ("Elapsed time (ms)"=w489:dbl, "error out"=w490:errorcluster)  [unwired: 5 in]
              n201 = Bundle("Elapsed time (ms)"=w489, "filename"=w476) -> (w488:T15)  [unwired: 1 in]
              n202 = Send Notification(notification=w488, notifier=w492) -> (notifier out=w491:refnum<notifier>)  [unwired: 1 in, 1 out]
            }
            frame True {
            }
          }
          n203 = Or(x=w468, y=w453) -> (x .or. y?=w470:bool)
          n204 = case shown="Error" w453 {
            tunnel: w455 -> [_ w473]
            tunnel: [_ w471] -> _
            frame No Error {
            }
            frame Error {
              n205 = Send Notification(notification=TRUE, notifier=w473) -> (error out=w471:errorcluster)  [unwired: 1 in, 1 out]
            }
          }
        }
        n206 = while {
          tunnel: w427 -> [w501]
          tunnel: w425 -> [w498]
          stop <- w500 stop-if-true
          # "STATUS"
          n207 = Wait on Notification(notifier=w501, ignore previous (F)=TRUE) -> (notification=w499:cluster{"elapsed":u32, "name":string}, error out=w500:errorcluster)  [unwired: 2 in, 2 out]
          n208 = case shown="No Error" w500 {
            tunnel: w499 -> [w509 _]
            tunnel: w498 -> [w508 _]
            frame No Error {
              n209 = Unbundle(w509) -> ("elapsed"=w504:u32, "name"=w503:string)
              n210 = Divide(x=w504, y=w508) -> (x/y=w505:dbl)
              n211 = Format Into String(format string="%d ms", w504) -> (resulting string=w506:string)  [unwired: 2 in, 1 out]
              n212 = local write "Status"(w503) -> ()
              n213 = property on="Load" class="Slide (strict)"("Value"=w505, "Caption.Text"=w506) -> ()  [unwired: 2 in, 2 out]
            }
            frame Error {
            }
          }
        }
        n214 = call "AIDI-Engine.vi"("Action"=AIDI-Action."Init & Start", "error in (no error)"=w416) -> ("error out"=w415:errorcluster)  [unwired: 8 in, 5 out]
        n215 = while {
          shift-right: [w446] -> w417
          shift-left: w415 -> [w451]
          tunnel: w411 -> [w440]
          shift-right: [w438] -> w409
          shift-left: w432 -> [w449]
          stop <- w447 stop-if-true
          # "PRODUCER"
          n216 = call "AIDI-Engine.vi"("Action"=AIDI-Action."Read", "error in (no error)"=w451) -> ("AI"=w444:dbl[][], "DI"=w443:bool[][], "error out"=w442:errorcluster)  [unwired: 8 in, 3 out]
          n217 = Bundle("AI"=w444, "DI"=w443) -> (w439:cluster{"AI":dbl[][], "DI":bool[][]})  [unwired: 1 in]
          n218 = Enqueue Element(queue=w440, element=w439, error in (no error)=w442) -> (error out=w441:errorcluster)  [unwired: 1 in, 2 out]
          n219 = Wait (ms)(milliseconds to wait=u32 5) -> ()  [unwired: 1 out]
          n220 = Wait on Notification(notifier=w449, timeout in ms (-1)=0, error in (no error)=w441) -> (notifier out=w438:refnum<notifier>, notification=w445:bool, error out=w446:errorcluster)  [unwired: 1 in, 1 out]
          n221 = Or(x=w446, y=w445) -> (x .or. y?=w447:bool)
        }
        n222 = call "AIDI-Engine.vi"("Action"=AIDI-Action."Clean up", "error in (no error)"=w417) -> ("error out"=w410:errorcluster)  [unwired: 8 in, 5 out]
        n223 = case shown="Error" w410 {
          selector: w410 -> [w433 w435]
          tunnel: w409 -> [_ w437]
          tunnel: [w433 w435] -> w408
          tunnel: [_ w434] -> _
          frame No Error {
          }
          frame Error {
            n224 = Send Notification(notification=TRUE, notifier=w437) -> (error out=w434:errorcluster)  [unwired: 1 in, 1 out]
          }
        }
        n225 = Merge Errors(w408, w420) -> (w421:errorcluster)
        n226 = call "Tosca-Clean Up AI Processing.vi"("state"=w419) -> ()  [unwired: 15 in]
        n227 = Release Notifier(notifier=w426) -> ()  [unwired: 2 in, 3 out]
        n228 = property on="finished" class="Clust (strict)"("Val(Sgnl)"=w421) -> ()  [unwired: 2 in, 2 out]
      }
      frame Error {
        n229 = Release Queue(queue=w510) -> ()  [unwired: 2 in, 3 out]
      }
    }
  }
  n230 = while {
    tunnel: w12 -> [w514]
    tunnel: w9 -> [w511]
    stop <- w513 stop-if-true
    # "IPC THREAD"
    n231 = Dequeue Element(queue=w514) -> (element=w512:cluster{"Action":string, "Data":variant}, error out=w513:errorcluster)  [unwired: 2 in, 2 out]
    n232 = case shown="No Error" w513 {
      tunnel: w512 -> [w518 _]
      tunnel: w511 -> [w515 _]
      frame No Error {
        n233 = Unbundle(w518) -> ("Action"=w517:string, "Data"=w516:variant)
        n234 = case shown="\"Run\"" w517 {
          tunnel: w516 -> [_ w522]
          tunnel: w515 -> [_ w524]
          frame "", Default {
          }
          frame "Run" {
            n235 = Unbundle By Name(w524) -> ("Run"=w523:refnum<user-event>)
            n236 = Variant To Data(type=T4 {"active"=FALSE, "Fs"=0.0, "AI"=[], "DI"=[]} ("AI"), Variant=w522) -> (data=w520:T4)  [unwired: 1 in, 1 out]
            n237 = Bundle("AI"=w520) -> (w519:cluster{"AI":T4})  [unwired: 1 in]
            n238 = Generate User Event(user event=w523, event data cluster=w519) -> ()  [unwired: 2 in, 2 out]
          }
        }
      }
      frame Error {
      }
    }
  }
  n239 = while {
    tunnel: w7 -> [w536]
    tunnel: w6 -> [w535]
    shift-right: [w527] -> _
    shift-left: w1 -> [w534]
    tunnel: w9 -> [w525]
    stop <- w526 stop-if-true
    # "TCP THREAD"
    n240 = while {
      tunnel: w536 -> [w593]
      tunnel: w535 -> [w592]
      shift-right: [w588] -> w533
      shift-left: w534 -> [w591]
      tunnel: [w589] -> w532
      tunnel: [w590] -> w531
      stop <- w587 stop-if-true
      n241 = call "TCP Generic Listener.vi"("net address"=w593, "port"=w592, "error in (no error)"=w591) -> ("connection ID"=w590:refnum<k5>, "Connected?"=w589:bool, "error out"=w588:errorcluster)  [unwired: 10 in]
      n242 = Or(x=w589, y=w588) -> (x .or. y?=w587:bool)
    }
    n243 = case shown="True" w532 {
      tunnel: w533 -> [w538 w549]
      tunnel: w531 -> [w539 w550]
      tunnel: [w539 w543] -> w529
      tunnel: [w538 w542] -> w528
      tunnel: [_ w541] -> w526
      tunnel: w525 -> [_ w540]
      frame False {
      }
      frame True {
        n244 = call "TCP Generic Grab Data.vi"("connection ID"=w550, "error in (no error)"=w549) -> ("connection ID out"=w546:refnum<k5>, "data out"=w548:string, "error out"=w547:errorcluster)  [unwired: 11 in]
        n245 = case shown="No Error" w547 {
          selector: w547 -> [_ w585]
          tunnel: w548 -> [w561 _]
          tunnel: w546 -> [w560 w586]
          tunnel: [w557 w586] -> w545
          tunnel: [w556 w585] -> w544
          tunnel: [w555 _] -> w541
          tunnel: w540 -> [w551 _]
          frame No Error {
            n246 = call "Parse String Fields.vi"("Separator"=";", "String"=w561) -> ("Fields"=w559:string[])  [unwired: 8 in, 1 out]
            n247 = Index Array(array=w559) -> (element #1=w558:string, element #2=w554:string, element #3=w553:string)  [unwired: 3 in]
            n248 = case shown="\"Quit\"" w558 {
              tunnel: w560 -> [w562 w569 w576 w580 w584]
              tunnel: [w562 w569 w576 w582 w584] -> w557
              tunnel: [_ w568 w575 w581 _] -> w556
              tunnel: [_ _ _ _ TRUE] -> w555
              tunnel: w554 -> [_ w565 _ _ _]
              tunnel: w553 -> [_ _ _ _ _]
              tunnel: w551 -> [_ w567 w574 _ _]
              frame "", Default {
              }
              frame "Start stream" {
                n249 = Unbundle By Name(w567) -> ("Record"=w566:refnum<user-event>)
                n250 = Bundle(TRUE, "Tag"=w565) -> (w564:cluster{bool, "Tag":string})  [unwired: 1 in]
                n251 = Generate User Event(user event=w566, event data cluster=w564) -> (error out=w568:errorcluster)  [unwired: 2 in, 1 out]
              }
              frame "Stop stream" {
                n252 = Unbundle By Name(w574) -> ("Record"=w573:refnum<user-event>)
                n253 = Bundle(FALSE, "") -> (w572:cluster{bool, string})  [unwired: 1 in]
                n254 = Generate User Event(user event=w573, event data cluster=w572) -> (error out=w575:errorcluster)  [unwired: 2 in, 1 out]
              }
              frame "Status" {
                n255 = local read "recording"() -> (w577:bool)
                n256 = Boolean To (0,1)(Boolean=w577) -> (0, 1=w578:i16)
                n257 = Type Cast(x=w578) -> (*(type *) &x=w579:string)  [unwired: 1 in]
                n258 = TCP Write(connection ID=w580, data in=w579) -> (connection ID out=w582:refnum<k5>, error out=w581:errorcluster)  [unwired: 2 in, 1 out]
              }
              frame "Quit" {
              }
            }
          }
          frame Error {
          }
        }
        n259 = call "TCP Generic Ack.vi"("error in (no error)"=w544, "connection ID"=w545) -> ("error out"=w542:errorcluster, "connection ID out"=w543:refnum<k5>)  [unwired: 8 in]
      }
    }
    n260 = Not A Number/Path/Refnum?(number/path/refnum=w529) -> (NaN/Path/Refnum?=w530:bool)
    n261 = case shown="False" w530 {
      tunnel: w529 -> [w537 _]
      frame False {
        n262 = TCP Close Connection(connection ID=w537) -> ()  [unwired: 2 in, 2 out]
      }
      frame True {
      }
    }
    n263 = call "Error Handler.vi"("error in (no error)"=w528) -> ("No Error"=w527:errorcluster)  [unwired: 12 in, 2 out]
  }
